vi "TrafficLight.vi"() -> ()   [LabVIEW 2015]
panel:
  in  "Car Waiting NS":bool
  in  "Car Waiting EW":bool
  in  "Light Time":sgl(slide)=1.0 min=1 max=30 step=1 scale=1.0..30.0
  in  "Flashing Red":bool
  in  "Emergency":bool
  out "NS2 G":bool
  out "NS2 Y":bool
  out "NS2 R":bool
  out "EW2 G":bool
  out "EW2 Y":bool
  out "EW2 R":bool
  out "NS1 G":bool
  out "NS1 Y":bool
  out "NS1 R":bool
  out "EW1 G":bool
  out "EW1 Y":bool
  out "EW1 R":bool
  in  "stop":bool
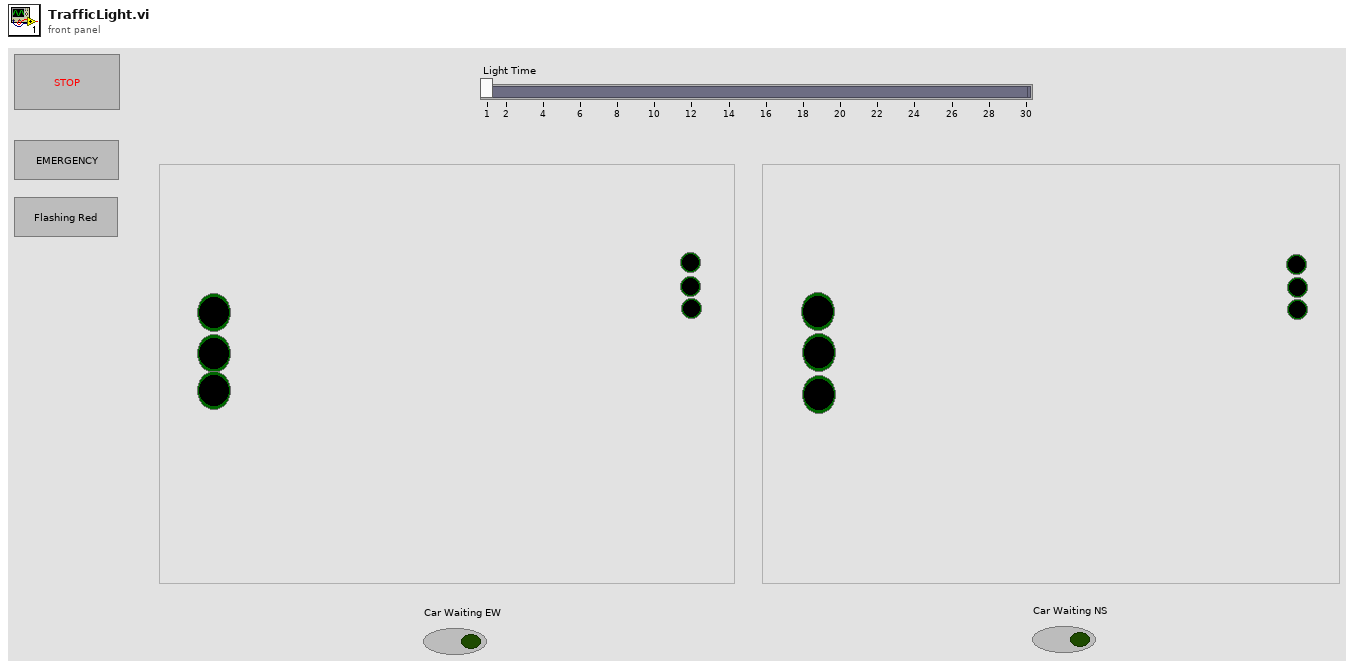
[diagram p1: front panel]
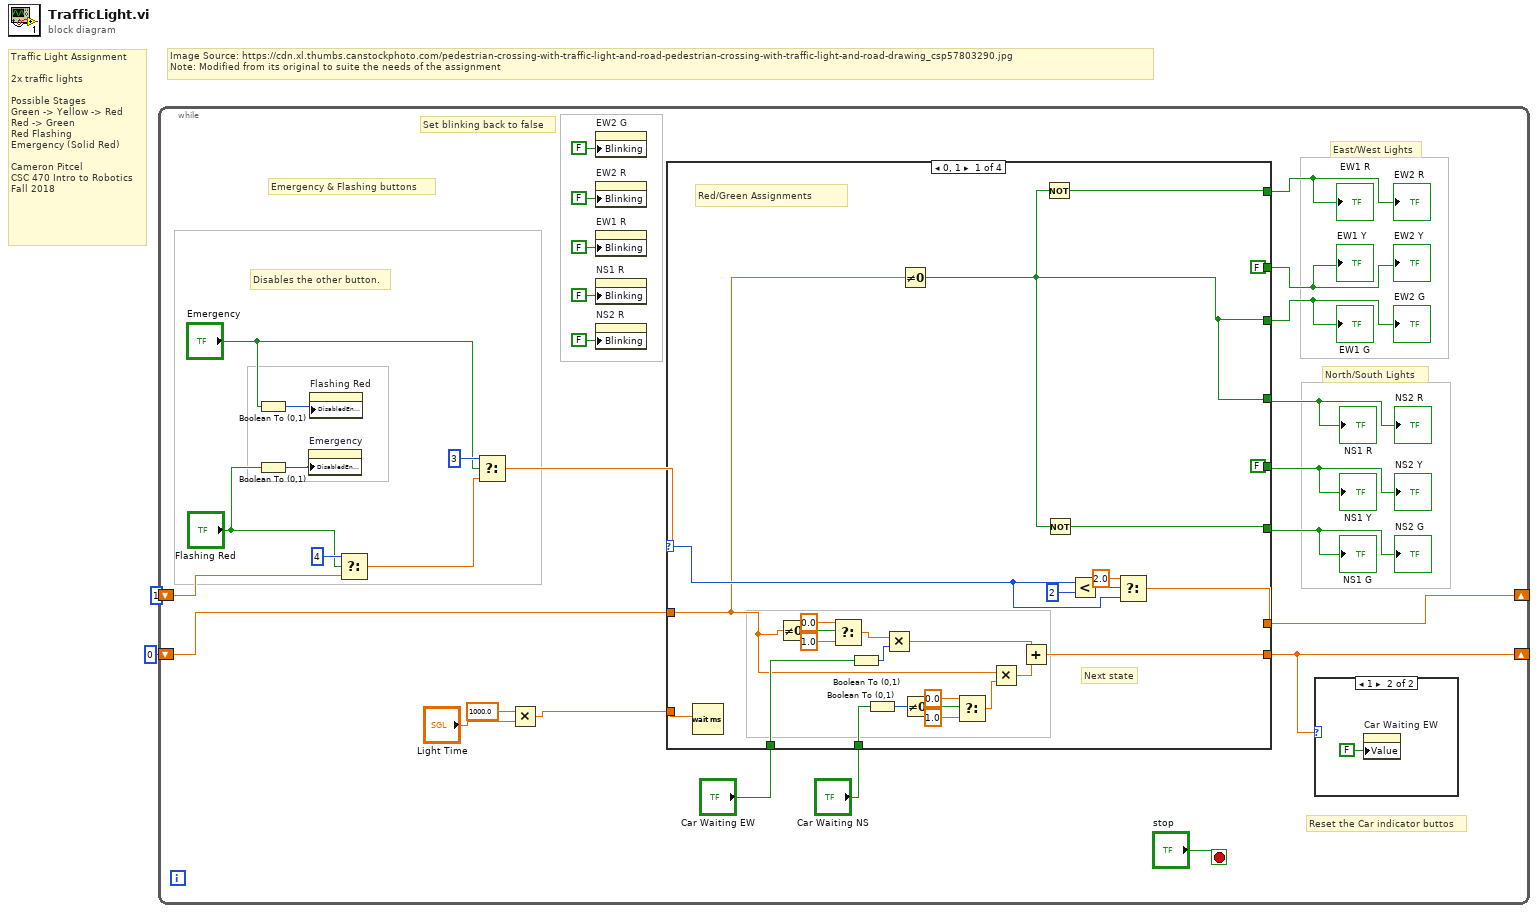
[diagram p0: block diagram]
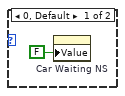
[diagram p2: hidden frame]
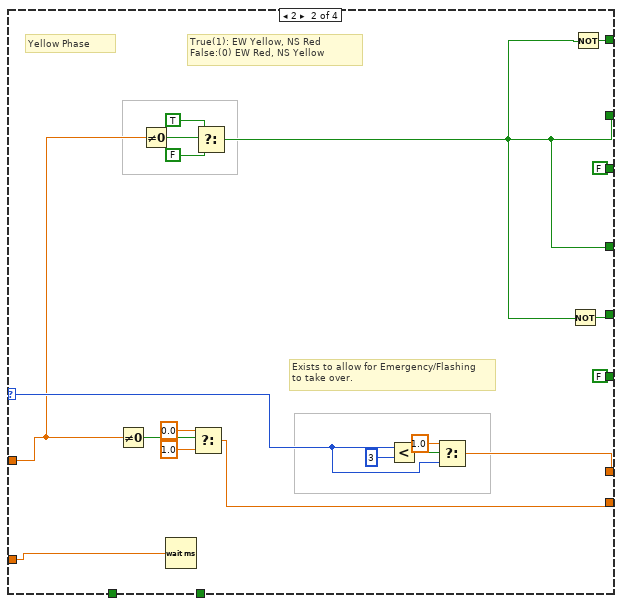
[diagram p3: hidden frame]
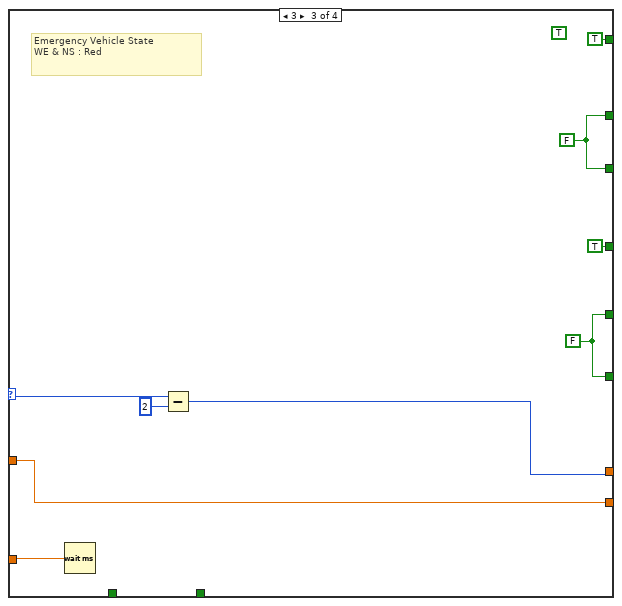
[diagram p4: hidden frame]
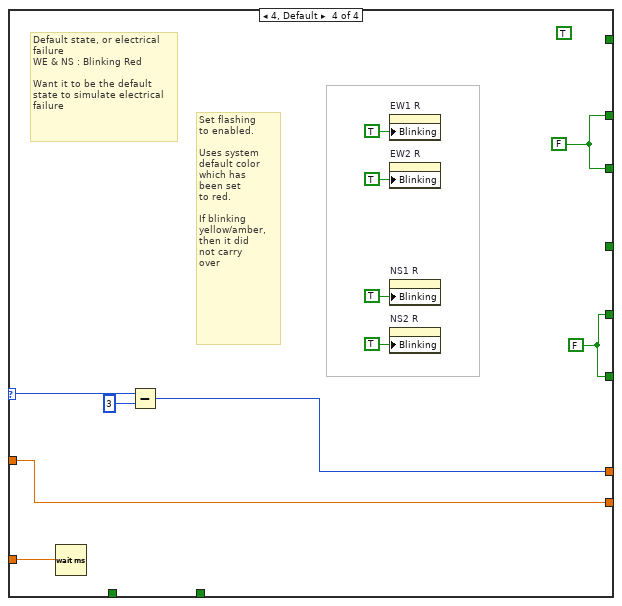
[diagram p5: hidden frame]
diagram:
  # "Image Source: https://cdn.xl.thumbs.canstockphoto.com/pedestrian-crossing-with-traffic-light-and-road-pedestrian-crossing-with-traffic-light-and-road-drawing_csp57803290.jpg\nNote: Modified from its original to suite the needs of the assignment"
  # "Traffic Light Assignment\n\n2x traffic lights\n\nPossible Stages\nGreen -> Yellow -> Red\nRed -> Green\nRed Flashing\nEmergency (Solid Red)\n\nCameron Pitcel\nCSC 470 Intro to Robotics\nFall 2018"
  n1 = while {
    shift-right: [w30] -> _
    shift-left: 1 -> [w23]
    shift-right: [w6] -> _
    shift-left: 0 -> [w7]
    stop <- "stop" stop-if-true
    # "Emergency & Flashing buttons"
    # "North/South Lights"
    # "East/West Lights"
    # "Reset the Car indicator buttos"
    # "Set blinking back to false"
    # "Disables the other button."
    n2 = Boolean To (0,1)(Boolean="Emergency") -> (0, 1=w17:i16)
    n3 = Boolean To (0,1)(Boolean="Flashing Red") -> (0, 1=w19:i16)
    n4 = property on="Emergency" class="Bool (strict)"("DisabledEnum"=w19) -> ()  [unwired: 2 in, 2 out]
    n5 = property on="Flashing Red" class="Bool (strict)"("DisabledEnum"=w17) -> ()  [unwired: 2 in, 2 out]
    n6 = Select(t=4, s="Flashing Red", f=w23) -> (s? t:f=w21:dbl)
    n7 = Select(t=3, s="Emergency", f=w21) -> (s? t:f=w18:dbl)
    n8 = Multiply(x=sgl 1000.0, y="Light Time") -> (x*y=w3:sgl)
    n9 = property on="EW2 G" class="Bool (strict)"("Blinking"=FALSE) -> ()  [unwired: 2 in, 2 out]
    n10 = property on="EW2 R" class="Bool (strict)"("Blinking"=FALSE) -> ()  [unwired: 2 in, 2 out]
    n11 = property on="EW1 R" class="Bool (strict)"("Blinking"=FALSE) -> ()  [unwired: 2 in, 2 out]
    n12 = property on="NS1 R" class="Bool (strict)"("Blinking"=FALSE) -> ()  [unwired: 2 in, 2 out]
    n13 = property on="NS2 R" class="Bool (strict)"("Blinking"=FALSE) -> ()  [unwired: 2 in, 2 out]
    n14 = case shown="0, 1" w18 {
      selector: w18 -> [w45 w76 w84 w97]
      tunnel: [w38 FALSE w86 w99] -> w27
      tunnel: [FALSE w62 w86 w99] -> w28
      tunnel: [w39 w65 TRUE _] -> w29
      tunnel: [w38 w62 TRUE _] -> w26
      tunnel: [FALSE w64 w85 w98] -> w25
      tunnel: [w37 FALSE w85 w98] -> w24
      tunnel: [w44 w75 w82 w95] -> w30
      tunnel: w3 -> [w60 w61 w81 w90]
      tunnel: "Car Waiting EW" -> [w35 _ _ _]
      tunnel: "Car Waiting NS" -> [w36 _ _ _]
      tunnel: w7 -> [w34 w70 w80 w89]
      tunnel: [w51 w72 w80 w89] -> w6
      frame 0, 1 {
        # "Next state"
        # "Red/Green Assignments"
        n15 = Wait (ms)(milliseconds to wait=w60) -> ()  [unwired: 1 out]
        n16 = Not Equal To 0?(x=w34) -> (x != 0?=w43:bool)
        n17 = Select(t=0.0, s=w43, f=1.0) -> (s? t:f=w40:dbl)
        n18 = Boolean To (0,1)(Boolean=w35) -> (0, 1=w59:i16)
        n19 = Boolean To (0,1)(Boolean=w36) -> (0, 1=w55:i16)
        n20 = Multiply(x=w40, y=w59) -> (x*y=w53:dbl)
        n21 = Not Equal To 0?(x=w34) -> (x != 0?=w38:bool)
        n22 = Not Equal To 0?(x=w55) -> (x != 0?=w58:bool)
        n23 = Select(t=0.0, s=w58, f=1.0) -> (s? t:f=w54:dbl)
        n24 = Multiply(x=w34, y=w54) -> (x*y=w52:dbl)
        n25 = Add(x=w53, y=w52) -> (x+y=w51:dbl)
        n26 = Not(x=w38) -> (.not. x?=w39:bool)
        n27 = Not(x=w38) -> (.not. x?=w37:bool)
        n28 = Less?(x=w45, y=2) -> (x < y?=w47:bool)
        n29 = Select(t=2.0, s=w47, f=w45) -> (s? t:f=w44:dbl)
      }
      frame 2 {
        # "Exists to allow for Emergency/Flashing\nto take over."
        # "True(1): EW Yellow, NS Red\nFalse:(0) EW Red, NS Yellow"
        # "Yellow Phase"
        n30 = Not Equal To 0?(x=w70) -> (x != 0?=w63:bool)
        n31 = Not Equal To 0?(x=w70) -> (x != 0?=w71:bool)
        n32 = Wait (ms)(milliseconds to wait=w61) -> ()  [unwired: 1 out]
        n33 = Select(t=0.0, s=w63, f=1.0) -> (s? t:f=w72:dbl)
        n34 = Select(t=TRUE, s=w71, f=FALSE) -> (s? t:f=w62:bool)
        n35 = Less?(x=w76, y=3) -> (x < y?=w78:bool)
        n36 = Select(t=1.0, s=w78, f=w76) -> (s? t:f=w75:dbl)
        n37 = Not(x=w62) -> (.not. x?=w64:bool)
        n38 = Not(x=w62) -> (.not. x?=w65:bool)
      }
      frame 3 {
        (unwired) TRUE ("Boolean")
        w85 = FALSE
        w86 = FALSE
        # "Emergency Vehicle State\nWE & NS : Red"
        n39 = Wait (ms)(milliseconds to wait=w81) -> ()  [unwired: 1 out]
        n40 = Subtract(x=w84, y=2) -> (x-y=w82:i32)
      }
      frame 4, Default {
        (unwired) TRUE ("Boolean")
        w98 = FALSE
        w99 = FALSE
        # "Set flashing\nto enabled.\n\nUses system\ndefault color\nwhich has\nbeen set\nto red.\n\nIf blinking \nyellow/amber,\nthen it did\nnot carry \nover"
        # "Default state, or electrical\nfailure\nWE & NS : Blinking Red\n\nWant it to be the default\nstate to simulate electrical\nfailure"
        n41 = Wait (ms)(milliseconds to wait=w90) -> ()  [unwired: 1 out]
        n42 = Subtract(x=w97, y=3) -> (x-y=w95:i32)
        n43 = property on="EW1 R" class="Bool (strict)"("Blinking"=TRUE) -> ()  [unwired: 2 in, 2 out]
        n44 = property on="EW2 R" class="Bool (strict)"("Blinking"=TRUE) -> ()  [unwired: 2 in, 2 out]
        n45 = property on="NS1 R" class="Bool (strict)"("Blinking"=TRUE) -> ()  [unwired: 2 in, 2 out]
        n46 = property on="NS2 R" class="Bool (strict)"("Blinking"=TRUE) -> ()  [unwired: 2 in, 2 out]
      }
    }
    "EW1 R" <- w29
    "NS2 Y" <- w25
    "NS2 G" <- w24
    "EW2 G" <- w27
    "EW2 R" <- w29
    "EW2 Y" <- w28
    "NS1 Y" <- w25
    "NS1 G" <- w24
    "NS2 R" <- w26
    "EW1 G" <- w27
    "EW1 Y" <- w28
    "NS1 R" <- w26
    n47 = case shown="1" w6 {
      frame 0, Default {
        n48 = property on="Car Waiting NS" class="Bool (strict)"("Value"=FALSE ("Car Waiting NS")) -> ()  [unwired: 2 in, 2 out]
      }
      frame 1 {
        n49 = property on="Car Waiting EW" class="Bool (strict)"("Value"=FALSE ("Car Waiting EW")) -> ()  [unwired: 2 in, 2 out]
      }
    }
  }
